vi "CRYSet Probe Waveform Front Panel.vi"(11 "Vi Ref":refnum<vi>) -> ()   [LabVIEW 2013]
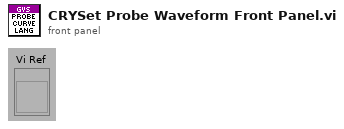
[diagram p1: front panel]
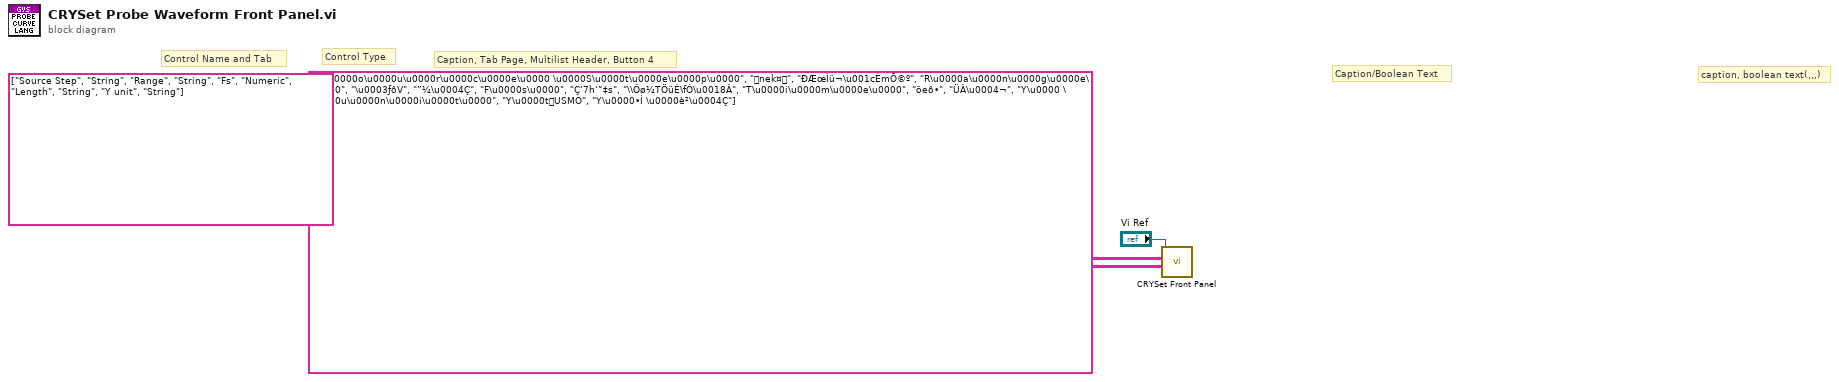
[diagram p0: block diagram]
diagram:
  # "Caption, Tab Page, Multilist Header, Button 4"
  # "Control Type"
  # "Control Name and Tab"
  # "caption, boolean text(,,,)"
  # "Caption/Boolean Text"
  n1 = call "CRYSet Front Panel.vi"("Caption(Boolean Text)"=string[][] [["S\u0000o\u0000u\u0000r\u0000c\u0000e\u0000 \u0000S\u0000t\u0000e\u0000p\u0000", "nek¤", "ÐÆœÌü¬\u001cÈmÕ©º"], ["R\u0000a\u0000n\u0000g\u0000e\u0000", "\u0003ƒôV", "”¼\u0004Ç"], ["F\u0000s\u0000", "Ç‘7h‘˜‡s", "\\Ôø¼TÖüÈ\fÓ\u0018Â"], ["T\u0000i\u0000m\u0000e\u0000", "öeô•", "ÜÂ\u0004¬"], ["Y\u0000 \u0000u\u0000n\u0000i\u0000t\u0000", "Y\u0000tUSMO", "Y\u0000•Í \u0000è²\u0004Ç"]], "Control ID and Type(Label Name, Type)"=string[][] [["Source Step", "String"], ["Range", "String"], ["Fs", "Numeric"], ["Length", "String"], ["Y unit", "String"]], "Vi Ref"="Vi Ref") -> ()  [unwired: 9 in]
